vi "Logic_Gate_Combination.vi"(1 "Array B":bool[](array[boolean]), 2 "Different Input Array Length Handle Flag":T1(ring), 3 "Boolean Operation Type":enum16{"AND", "OR", "XOR"}(ring), 4 "Array A":bool[](array[boolean])) -> (0 "Output Array":bool[](array[boolean]))   [LabVIEW 2015]
doc: "Help by FRC Team 836 - The RoboBees\n\nThis VI is a good trainer on how AND, OR, and XOR Boolean functions operate.\nThe user selects which Boolean to use.\n\"True\" values are loaded into the input arrays by clicking the buttons for Array A & B.\nThe output array will display the Boolean operation result.\nThe \"Different Input Array Length\" flag instructs how the VI handles situatioons where the input arrays are not the same size.\n\nNote: the arrays do not reset while in operation OR after restarting. The arrays must be reset using the \"Reinitialize to default\" operation\nin the \"Edit\" menu."
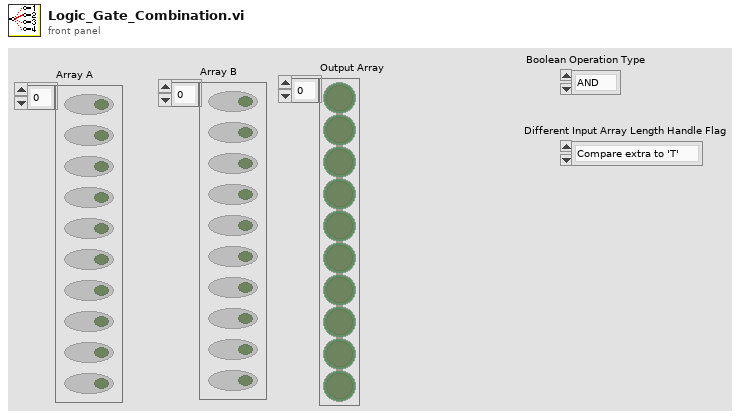
[diagram p1: front panel]
types:
  T1 = enum16{"Compare extra to 'T'", "Compare extra to 'F'", "Add extra to end"}
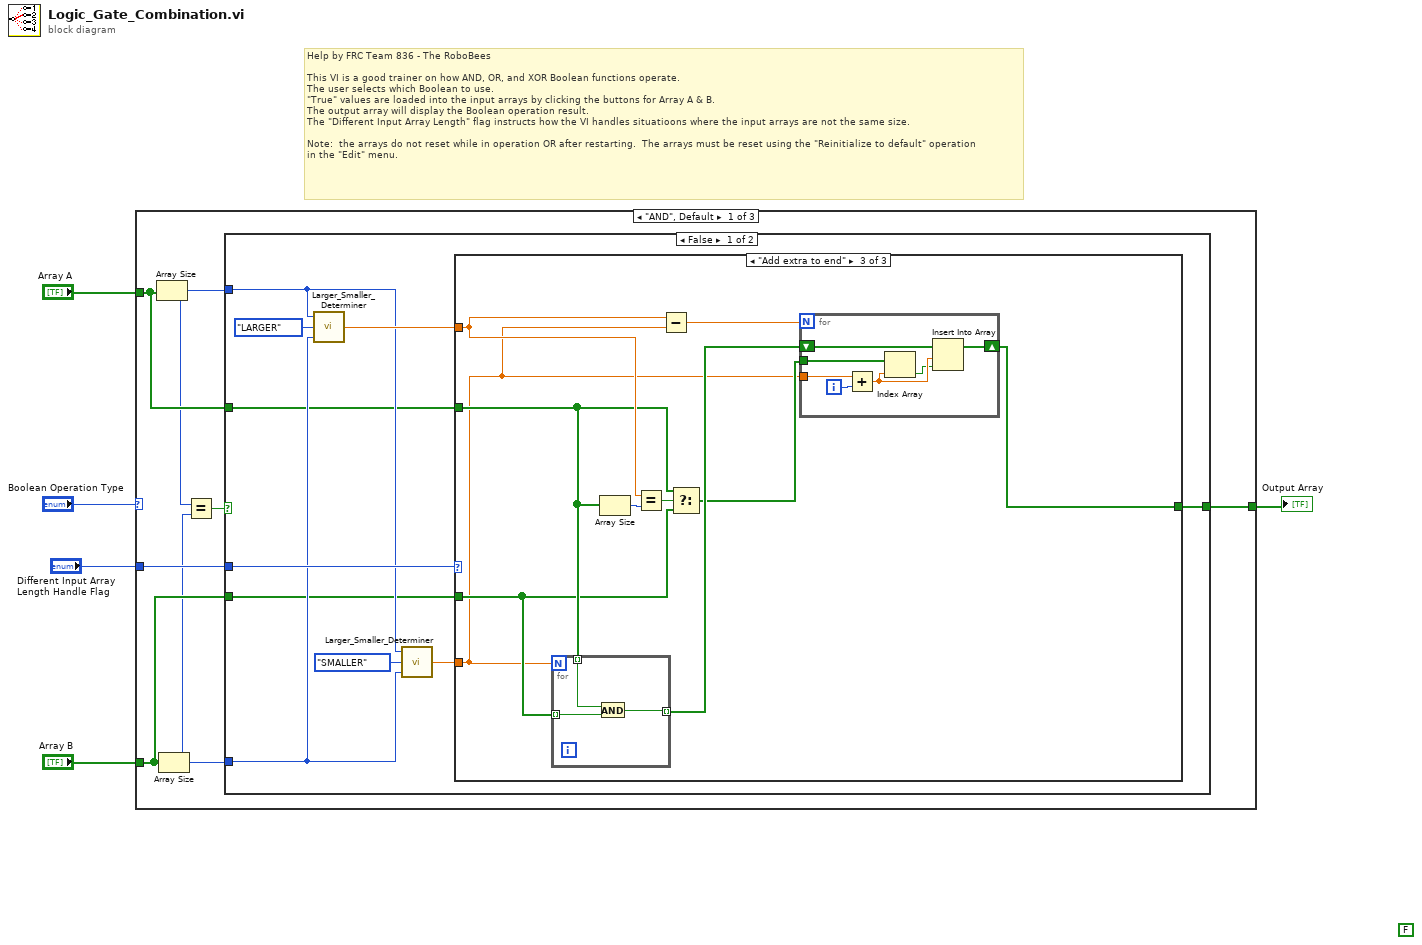
[diagram p0: block diagram]
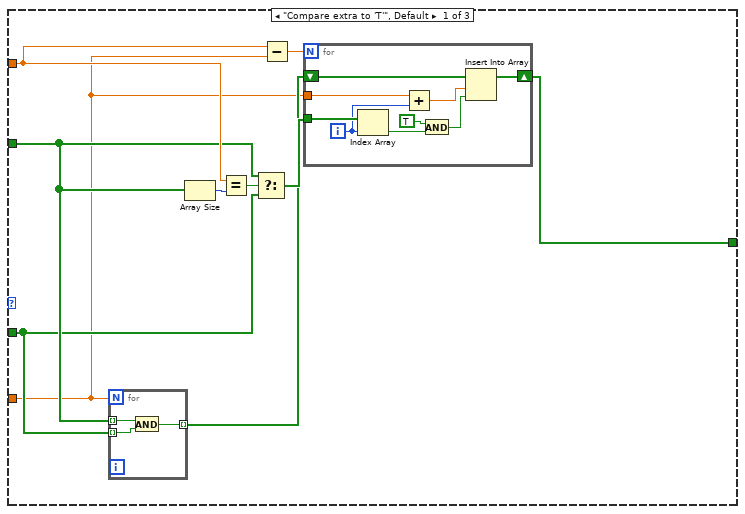
[diagram p2: hidden frame]
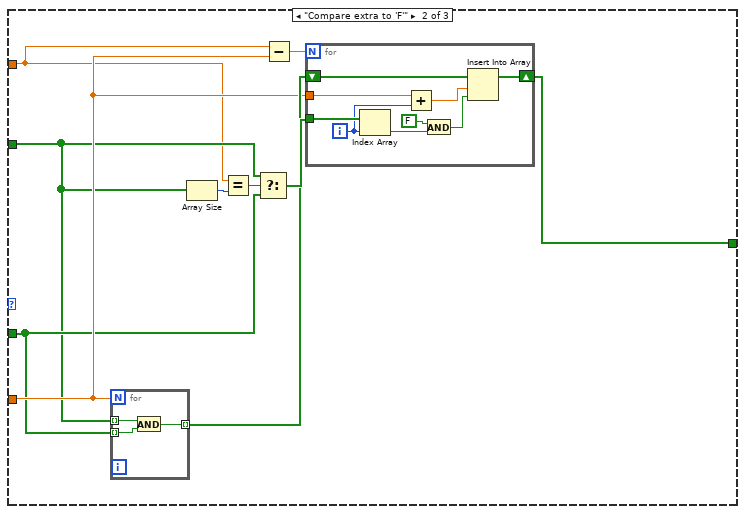
[diagram p3: hidden frame]
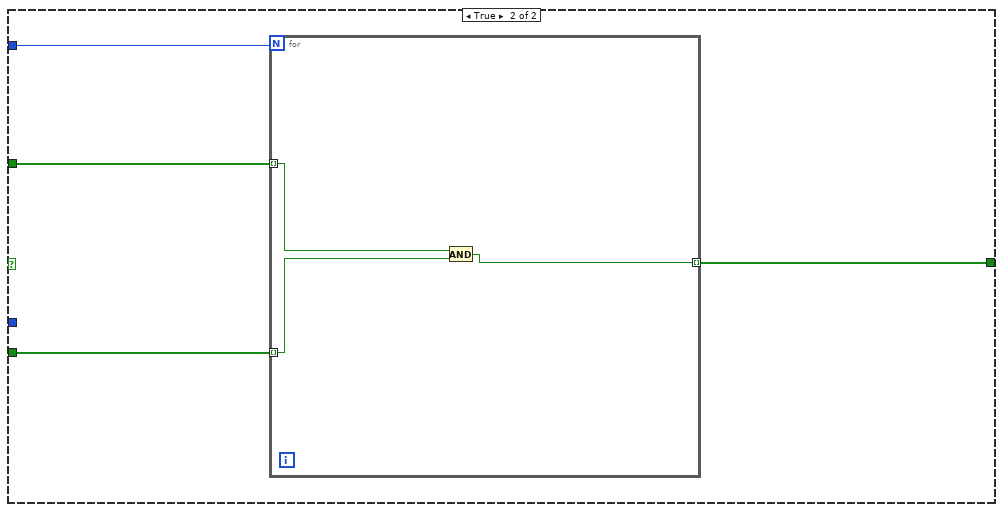
[diagram p4: hidden frame]
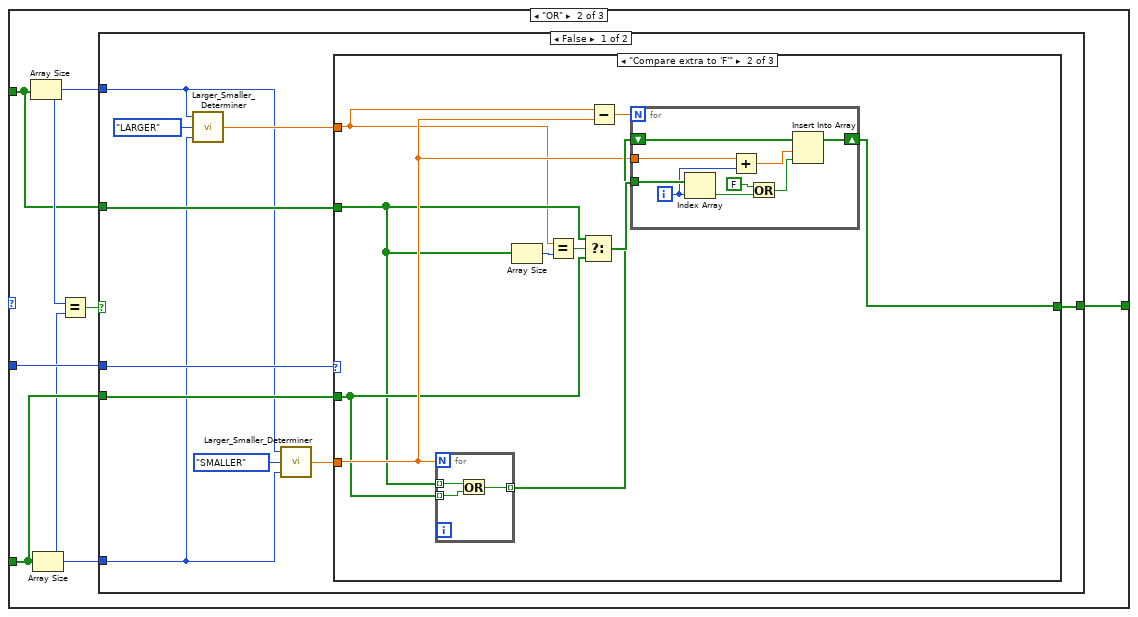
[diagram p5: hidden frame]
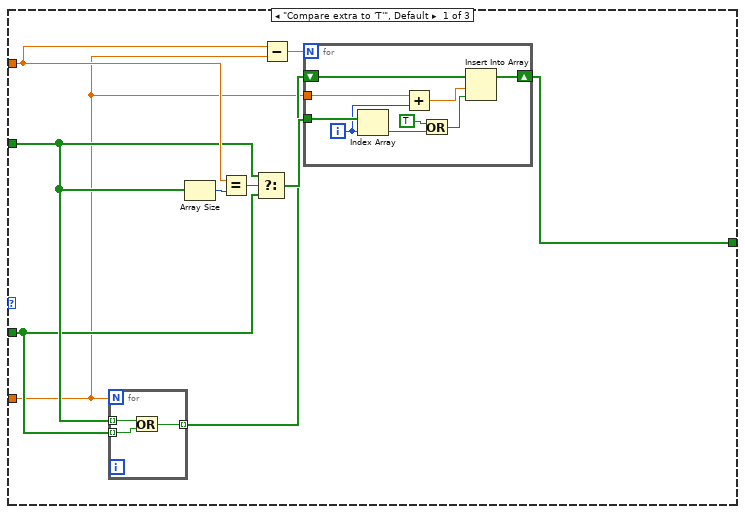
[diagram p6: hidden frame]
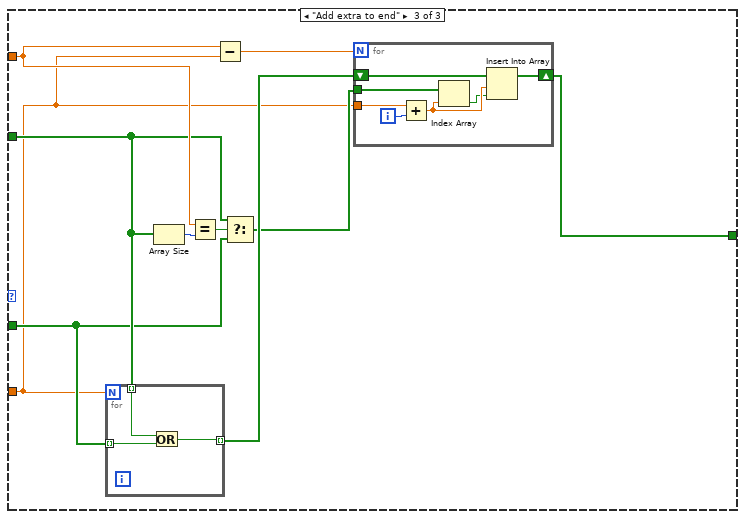
[diagram p7: hidden frame]
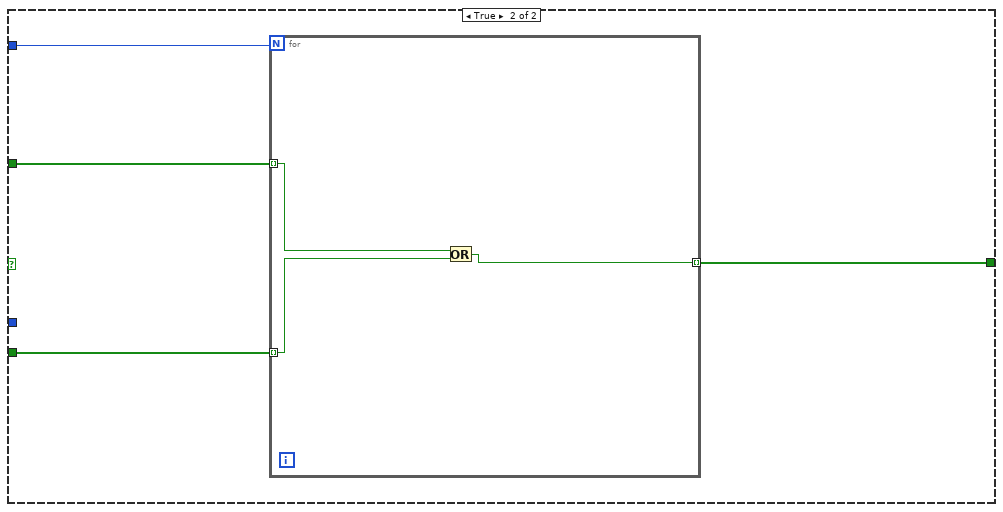
[diagram p8: hidden frame]
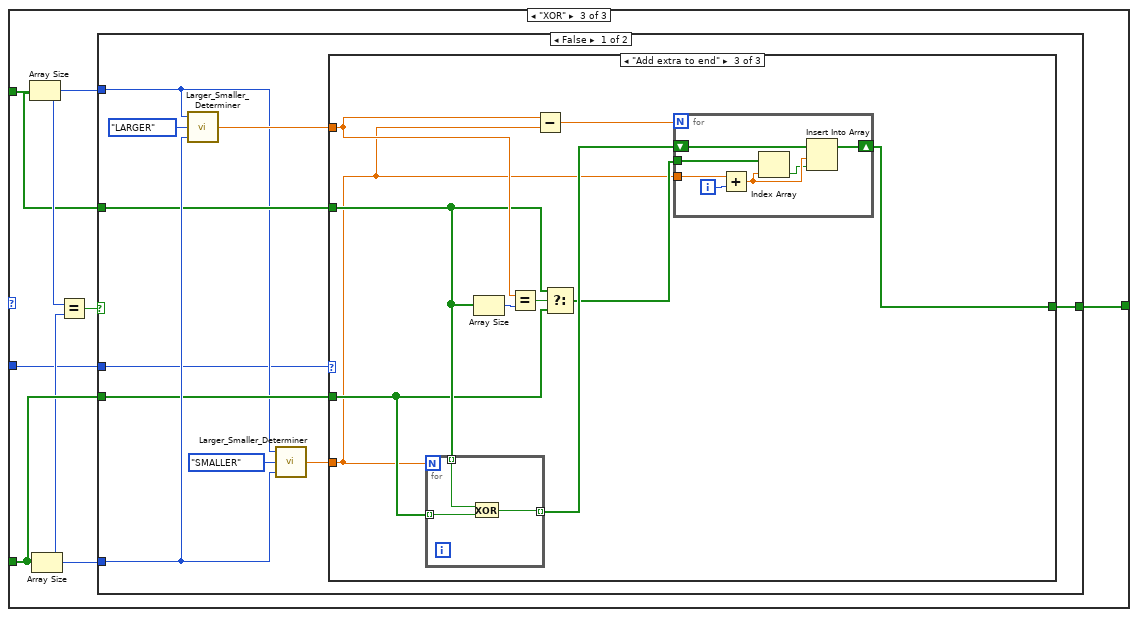
[diagram p9: hidden frame]
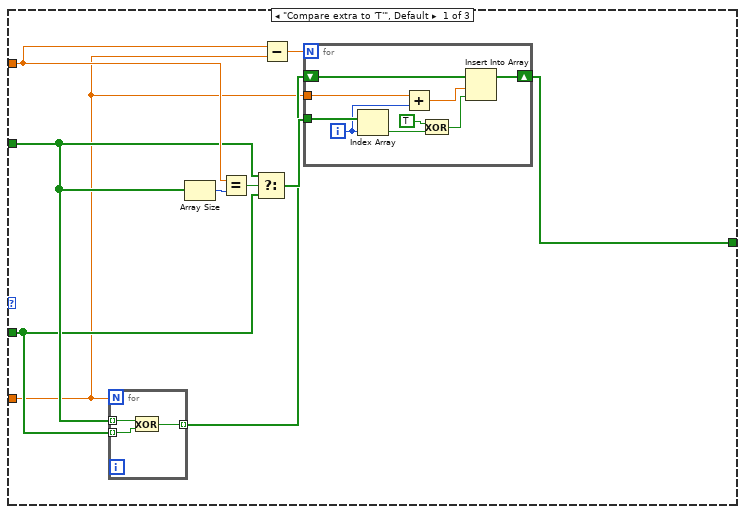
[diagram p10: hidden frame]
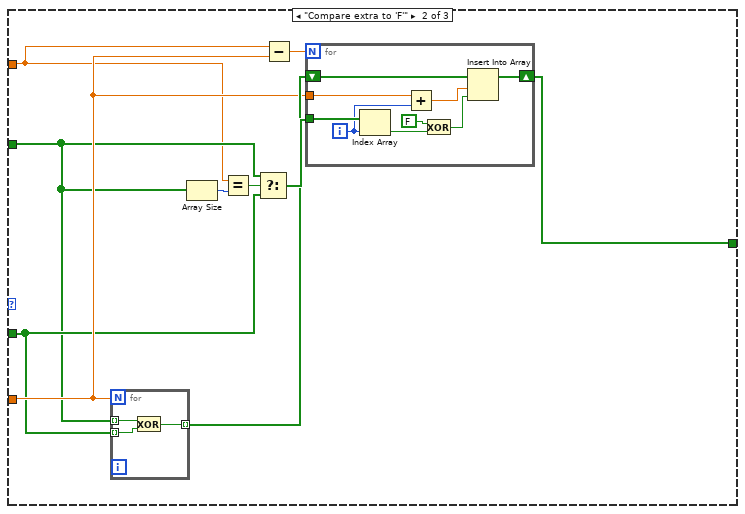
[diagram p11: hidden frame]
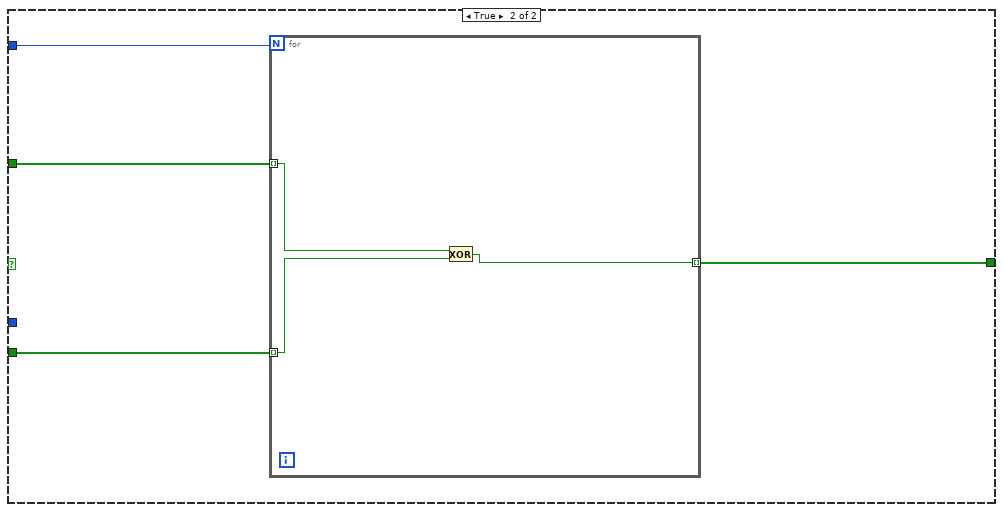
[diagram p12: hidden frame]
diagram:
  (unwired) FALSE
  # "Help by FRC Team 836 - The RoboBees\n\nThis VI is a good trainer on how AND, OR, and XOR Boolean functions operate.\nThe user selects which Boolean to use.\n\"True\" values are loaded into the input arrays by clicking the buttons for Array A & B.\nThe output array will display the Boolean operation result.\nThe \"Different Input Array Length\" flag instructs how the VI handles situatioons where the input arrays are not the same size.\n\nNote:  the arrays do not reset while in operation OR after restarting.  The arrays must be reset using the \"Reinitialize to default\" operation\nin the \"Edit\" menu."
  n1 = case shown="\"AND\", Default" "Boolean Operation Type" {
    tunnel: "Array A" -> [w11 w97 w186]
    tunnel: "Array B" -> [w10 w98 w185]
    tunnel: [w8 w96 w184] -> w2
    tunnel: "Different Input Array Length Handle Flag" -> [w7 w95 w182]
    frame "AND", Default {
      n2 = Array Size(array=w11) -> (size(s)=w9:i32)
      n3 = Array Size(array=w10) -> (size(s)=w6:i32)
      n4 = Equal?(x=w9, y=w6) -> (x = y?=w12:bool)
      n5 = case shown="False" w12 {
        tunnel: w11 -> [w16 w90]
        tunnel: w10 -> [w15 w89]
        tunnel: w9 -> [w18 w88]
        tunnel: [w13 w87] -> w8
        tunnel: w7 -> [w21 _]
        tunnel: w6 -> [w19 _]
        frame False {
          n6 = call <userlib>:"Larger_Smaller_Determiner.vi"("Input B"=w19, "Get Flag"=enum16{"LARGER", "SMALLER"}."LARGER", "Input A"=w18) -> ("Output Number"=w22:dbl)
          n7 = call <userlib>:"Larger_Smaller_Determiner.vi"("Input B"=w19, "Get Flag"=enum16{"LARGER", "SMALLER"}."SMALLER", "Input A"=w18) -> ("Output Number"=w17:dbl)
          n8 = case shown="\"Add extra to end\"" w21 {
            tunnel: w22 -> [w28 w46 w72]
            tunnel: w17 -> [w24 w49 w68]
            tunnel: w16 -> [w27 w47 w71]
            tunnel: w15 -> [w26 w48 w70]
            tunnel: [w23 w45 w67] -> w13
            frame "Compare extra to 'T'", Default {
              n9 = for {
                N: w24 -> [_]
                tunnel: w27 -> [w44] mode=indexing
                tunnel: w26 -> [w43] mode=indexing
                tunnel: [w42] -> w25 mode=indexing
                n10 = And(x=w44, y=w43) -> (x .and. y?=w42:bool)
              }
              n11 = Array Size(array=w27) -> (size(s)=w29:i32)
              n12 = Equal?(x=w28, y=w29) -> (x = y?=w30:bool)
              n13 = Select(t=w27, s=w30, f=w26) -> (s? t:f=w31:bool[])
              n14 = Subtract(x=w28, y=w24) -> (x-y=w32:dbl)
              n15 = for {
                N: w32 -> [_]
                tunnel: w31 -> [w37]
                shift-right: [w41] -> w23
                shift-left: w25 -> [w40]
                tunnel: w24 -> [w39]
                i -> [w34]
                n16 = Index Array(array=w37, index=w34) -> (element=w36:bool)
                n17 = Add(x=w39, y=w34) -> (x+y=w38:dbl)
                n18 = And(x=TRUE, y=w36) -> (x .and. y?=w33:bool)
                n19 = Insert Into Array(array=w40, index=w38, new element=w33) -> (w41:bool[])
              }
            }
            frame "Compare extra to 'F'" {
              n20 = for {
                N: w49 -> [_]
                tunnel: w47 -> [w66] mode=indexing
                tunnel: w48 -> [w65] mode=indexing
                tunnel: [w64] -> w50 mode=indexing
                n21 = And(x=w66, y=w65) -> (x .and. y?=w64:bool)
              }
              n22 = Array Size(array=w47) -> (size(s)=w51:i32)
              n23 = Equal?(x=w46, y=w51) -> (x = y?=w52:bool)
              n24 = Select(t=w47, s=w52, f=w48) -> (s? t:f=w53:bool[])
              n25 = Subtract(x=w46, y=w49) -> (x-y=w54:dbl)
              n26 = for {
                N: w54 -> [_]
                tunnel: w53 -> [w59]
                shift-right: [w63] -> w45
                shift-left: w50 -> [w62]
                tunnel: w49 -> [w61]
                i -> [w56]
                n27 = Index Array(array=w59, index=w56) -> (element=w58:bool)
                n28 = Add(x=w61, y=w56) -> (x+y=w60:dbl)
                n29 = And(x=FALSE, y=w58) -> (x .and. y?=w55:bool)
                n30 = Insert Into Array(array=w62, index=w60, new element=w55) -> (w63:bool[])
              }
            }
            frame "Add extra to end" {
              n31 = for {
                N: w68 -> [_]
                tunnel: w71 -> [w86] mode=indexing
                tunnel: w70 -> [w85] mode=indexing
                tunnel: [w84] -> w75 mode=indexing
                n32 = And(x=w86, y=w85) -> (x .and. y?=w84:bool)
              }
              n33 = Array Size(array=w71) -> (size(s)=w73:i32)
              n34 = Equal?(x=w72, y=w73) -> (x = y?=w74:bool)
              n35 = Subtract(x=w72, y=w68) -> (x-y=w76:dbl)
              n36 = Select(t=w71, s=w74, f=w70) -> (s? t:f=w69:bool[])
              n37 = for {
                N: w76 -> [_]
                tunnel: w69 -> [w81]
                tunnel: w68 -> [w82]
                shift-right: [w80] -> w67
                shift-left: w75 -> [w79]
                i -> [w83]
                n38 = Add(x=w82, y=w83) -> (x+y=w78:dbl)
                n39 = Index Array(array=w81, index=w78) -> (element=w77:bool)
                n40 = Insert Into Array(array=w79, index=w78, new element=w77) -> (w80:bool[])
              }
            }
          }
        }
        frame True {
          n41 = for {
            N: w88 -> [_]
            tunnel: w90 -> [w93] mode=indexing
            tunnel: w89 -> [w92] mode=indexing
            tunnel: [w91] -> w87 mode=indexing
            n42 = And(x=w93, y=w92) -> (x .and. y?=w91:bool)
          }
        }
      }
    }
    frame "OR" {
      n43 = Array Size(array=w97) -> (size(s)=w99:i32)
      n44 = Array Size(array=w98) -> (size(s)=w94:i32)
      n45 = Equal?(x=w99, y=w94) -> (x = y?=w100:bool)
      n46 = case shown="False" w100 {
        tunnel: w97 -> [w104 w178]
        tunnel: w98 -> [w106 w177]
        tunnel: w99 -> [w103 w176]
        tunnel: [w101 w175] -> w96
        tunnel: w95 -> [w105 _]
        tunnel: w94 -> [w102 _]
        frame False {
          n47 = call <userlib>:"Larger_Smaller_Determiner.vi"("Input B"=w102, "Get Flag"=enum16{"LARGER", "SMALLER"}."LARGER", "Input A"=w103) -> ("Output Number"=w110:dbl)
          n48 = call <userlib>:"Larger_Smaller_Determiner.vi"("Input B"=w102, "Get Flag"=enum16{"LARGER", "SMALLER"}."SMALLER", "Input A"=w103) -> ("Output Number"=w108:dbl)
          n49 = case shown="\"Compare extra to 'F'\"" w105 {
            tunnel: w110 -> [w116 w134 w160]
            tunnel: w108 -> [w112 w137 w156]
            tunnel: w104 -> [w115 w135 w159]
            tunnel: w106 -> [w114 w136 w158]
            tunnel: [w111 w133 w155] -> w101
            frame "Compare extra to 'T'", Default {
              n50 = for {
                N: w112 -> [_]
                tunnel: w115 -> [w132] mode=indexing
                tunnel: w114 -> [w131] mode=indexing
                tunnel: [w130] -> w113 mode=indexing
                n51 = Or(x=w132, y=w131) -> (x .or. y?=w130:bool)
              }
              n52 = Array Size(array=w115) -> (size(s)=w117:i32)
              n53 = Equal?(x=w116, y=w117) -> (x = y?=w118:bool)
              n54 = Select(t=w115, s=w118, f=w114) -> (s? t:f=w119:bool[])
              n55 = Subtract(x=w116, y=w112) -> (x-y=w120:dbl)
              n56 = for {
                N: w120 -> [_]
                tunnel: w119 -> [w125]
                shift-right: [w129] -> w111
                shift-left: w113 -> [w128]
                tunnel: w112 -> [w127]
                i -> [w122]
                n57 = Index Array(array=w125, index=w122) -> (element=w124:bool)
                n58 = Add(x=w127, y=w122) -> (x+y=w126:dbl)
                n59 = Or(x=TRUE, y=w124) -> (x .or. y?=w121:bool)
                n60 = Insert Into Array(array=w128, index=w126, new element=w121) -> (w129:bool[])
              }
            }
            frame "Compare extra to 'F'" {
              n61 = for {
                N: w137 -> [_]
                tunnel: w135 -> [w154] mode=indexing
                tunnel: w136 -> [w153] mode=indexing
                tunnel: [w152] -> w138 mode=indexing
                n62 = Or(x=w154, y=w153) -> (x .or. y?=w152:bool)
              }
              n63 = Array Size(array=w135) -> (size(s)=w139:i32)
              n64 = Equal?(x=w134, y=w139) -> (x = y?=w140:bool)
              n65 = Select(t=w135, s=w140, f=w136) -> (s? t:f=w141:bool[])
              n66 = Subtract(x=w134, y=w137) -> (x-y=w142:dbl)
              n67 = for {
                N: w142 -> [_]
                tunnel: w141 -> [w147]
                shift-right: [w151] -> w133
                shift-left: w138 -> [w150]
                tunnel: w137 -> [w149]
                i -> [w144]
                n68 = Index Array(array=w147, index=w144) -> (element=w146:bool)
                n69 = Add(x=w149, y=w144) -> (x+y=w148:dbl)
                n70 = Or(x=FALSE, y=w146) -> (x .or. y?=w143:bool)
                n71 = Insert Into Array(array=w150, index=w148, new element=w143) -> (w151:bool[])
              }
            }
            frame "Add extra to end" {
              n72 = for {
                N: w156 -> [_]
                tunnel: w159 -> [w174] mode=indexing
                tunnel: w158 -> [w173] mode=indexing
                tunnel: [w172] -> w163 mode=indexing
                n73 = Or(x=w174, y=w173) -> (x .or. y?=w172:bool)
              }
              n74 = Array Size(array=w159) -> (size(s)=w161:i32)
              n75 = Equal?(x=w160, y=w161) -> (x = y?=w162:bool)
              n76 = Subtract(x=w160, y=w156) -> (x-y=w164:dbl)
              n77 = Select(t=w159, s=w162, f=w158) -> (s? t:f=w157:bool[])
              n78 = for {
                N: w164 -> [_]
                tunnel: w157 -> [w169]
                tunnel: w156 -> [w170]
                shift-right: [w168] -> w155
                shift-left: w163 -> [w167]
                i -> [w171]
                n79 = Add(x=w170, y=w171) -> (x+y=w166:dbl)
                n80 = Index Array(array=w169, index=w166) -> (element=w165:bool)
                n81 = Insert Into Array(array=w167, index=w166, new element=w165) -> (w168:bool[])
              }
            }
          }
        }
        frame True {
          n82 = for {
            N: w176 -> [_]
            tunnel: w178 -> [w181] mode=indexing
            tunnel: w177 -> [w180] mode=indexing
            tunnel: [w179] -> w175 mode=indexing
            n83 = Or(x=w181, y=w180) -> (x .or. y?=w179:bool)
          }
        }
      }
    }
    frame "XOR" {
      n84 = Array Size(array=w186) -> (size(s)=w187:i32)
      n85 = Array Size(array=w185) -> (size(s)=w183:i32)
      n86 = Equal?(x=w187, y=w183) -> (x = y?=w188:bool)
      n87 = case shown="False" w188 {
        tunnel: w186 -> [w192 w266]
        tunnel: w185 -> [w193 w265]
        tunnel: w187 -> [w191 w264]
        tunnel: [w189 w263] -> w184
        tunnel: w183 -> [w194 _]
        tunnel: w182 -> [w190 _]
        frame False {
          n88 = call <userlib>:"Larger_Smaller_Determiner.vi"("Input B"=w194, "Get Flag"=enum16{"LARGER", "SMALLER"}."LARGER", "Input A"=w191) -> ("Output Number"=w198:dbl)
          n89 = call <userlib>:"Larger_Smaller_Determiner.vi"("Input B"=w194, "Get Flag"=enum16{"LARGER", "SMALLER"}."SMALLER", "Input A"=w191) -> ("Output Number"=w196:dbl)
          n90 = case shown="\"Add extra to end\"" w190 {
            tunnel: w198 -> [w204 w222 w248]
            tunnel: w196 -> [w200 w225 w244]
            tunnel: w192 -> [w203 w223 w247]
            tunnel: w193 -> [w202 w224 w246]
            tunnel: [w199 w221 w243] -> w189
            frame "Compare extra to 'T'", Default {
              n91 = for {
                N: w200 -> [_]
                tunnel: w203 -> [w220] mode=indexing
                tunnel: w202 -> [w219] mode=indexing
                tunnel: [w218] -> w201 mode=indexing
                n92 = Exclusive Or(1:w219, 2:w220) -> (0:w218:bool)
              }
              n93 = Array Size(array=w203) -> (size(s)=w205:i32)
              n94 = Equal?(x=w204, y=w205) -> (x = y?=w206:bool)
              n95 = Select(t=w203, s=w206, f=w202) -> (s? t:f=w207:bool[])
              n96 = Subtract(x=w204, y=w200) -> (x-y=w208:dbl)
              n97 = for {
                N: w208 -> [_]
                tunnel: w207 -> [w213]
                shift-right: [w217] -> w199
                shift-left: w201 -> [w216]
                tunnel: w200 -> [w215]
                i -> [w210]
                n98 = Index Array(array=w213, index=w210) -> (element=w212:bool)
                n99 = Add(x=w215, y=w210) -> (x+y=w214:dbl)
                n100 = Exclusive Or(1:w212, 2:TRUE ("x")) -> (0:w209:bool)
                n101 = Insert Into Array(array=w216, index=w214, new element=w209) -> (w217:bool[])
              }
            }
            frame "Compare extra to 'F'" {
              n102 = for {
                N: w225 -> [_]
                tunnel: w223 -> [w242] mode=indexing
                tunnel: w224 -> [w241] mode=indexing
                tunnel: [w240] -> w226 mode=indexing
                n103 = Exclusive Or(1:w241, 2:w242) -> (0:w240:bool)
              }
              n104 = Array Size(array=w223) -> (size(s)=w227:i32)
              n105 = Equal?(x=w222, y=w227) -> (x = y?=w228:bool)
              n106 = Select(t=w223, s=w228, f=w224) -> (s? t:f=w229:bool[])
              n107 = Subtract(x=w222, y=w225) -> (x-y=w230:dbl)
              n108 = for {
                N: w230 -> [_]
                tunnel: w229 -> [w235]
                shift-right: [w239] -> w221
                shift-left: w226 -> [w238]
                tunnel: w225 -> [w237]
                i -> [w232]
                n109 = Index Array(array=w235, index=w232) -> (element=w234:bool)
                n110 = Add(x=w237, y=w232) -> (x+y=w236:dbl)
                n111 = Exclusive Or(1:w234, 2:FALSE ("x")) -> (0:w231:bool)
                n112 = Insert Into Array(array=w238, index=w236, new element=w231) -> (w239:bool[])
              }
            }
            frame "Add extra to end" {
              n113 = for {
                N: w244 -> [_]
                tunnel: w247 -> [w262] mode=indexing
                tunnel: w246 -> [w261] mode=indexing
                tunnel: [w260] -> w251 mode=indexing
                n114 = Exclusive Or(1:w261, 2:w262) -> (0:w260:bool)
              }
              n115 = Array Size(array=w247) -> (size(s)=w249:i32)
              n116 = Equal?(x=w248, y=w249) -> (x = y?=w250:bool)
              n117 = Subtract(x=w248, y=w244) -> (x-y=w252:dbl)
              n118 = Select(t=w247, s=w250, f=w246) -> (s? t:f=w245:bool[])
              n119 = for {
                N: w252 -> [_]
                tunnel: w245 -> [w257]
                tunnel: w244 -> [w258]
                shift-right: [w256] -> w243
                shift-left: w251 -> [w255]
                i -> [w259]
                n120 = Add(x=w258, y=w259) -> (x+y=w254:dbl)
                n121 = Index Array(array=w257, index=w254) -> (element=w253:bool)
                n122 = Insert Into Array(array=w255, index=w254, new element=w253) -> (w256:bool[])
              }
            }
          }
        }
        frame True {
          n123 = for {
            N: w264 -> [_]
            tunnel: w266 -> [w269] mode=indexing
            tunnel: w265 -> [w268] mode=indexing
            tunnel: [w267] -> w263 mode=indexing
            n124 = Exclusive Or(1:w268, 2:w269) -> (0:w267:bool)
          }
        }
      }
    }
  }
  "Output Array" <- w2
